vi "Write Measurement Cycles.vi"(8 "error in (no error)":errorcluster, 10 "measurement cycles":dbl=1.0, 11 "signal configuration":refnum<class "SV Function.lvclass">) -> (0 "error out":errorcluster, 3 "signal configuration":refnum<class "SV Function.lvclass">)   [LabVIEW 2017, in "SV Function.lvclass"]
uses:
  <vilib>/addons/_NISVFA/_Generation/Signal Generation/SV Function/SV Function.lvclass
  <vilib>/addons/_NISVFA/_Generation/Signal Generation/SV Function/SV Function.lvclass/SV Function.ctl
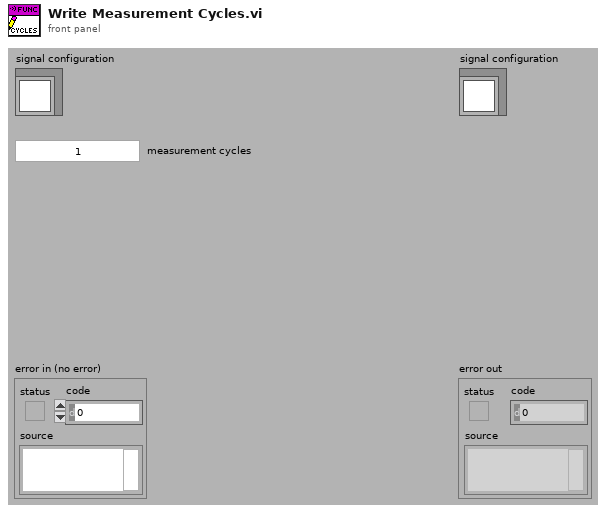
[diagram p1: front panel]
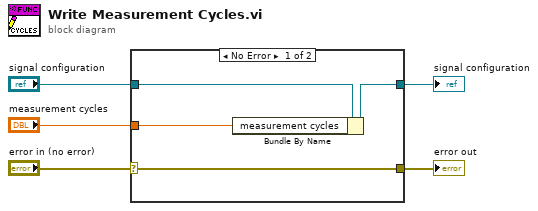
[diagram p0: block diagram]
diagram:
  n1 = case shown="No Error" "error in (no error)" {
    selector: "error in (no error)" -> [w9 w10]
    tunnel: [w9 w10] -> w4
    tunnel: [w7 w11] -> w2
    tunnel: "signal configuration" -> [w8 w11]
    tunnel: "measurement cycles" -> [w6 _]
    frame No Error {
      n2 = Bundle By Name(cluster=w8, "measurement cycles"=w6) -> (w7:refnum<class "SV Function.lvclass">)
    }
    frame Error {
    }
  }
  "error out" <- w4
  "signal configuration" <- w2
